vi "Decide Color Rank.vi"(11 "Numeric":dbl) -> (3 "Color Box":u32(colorbox))   [LabVIEW 2014]
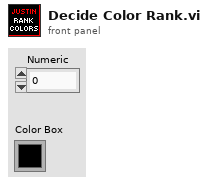
[diagram p1: front panel]
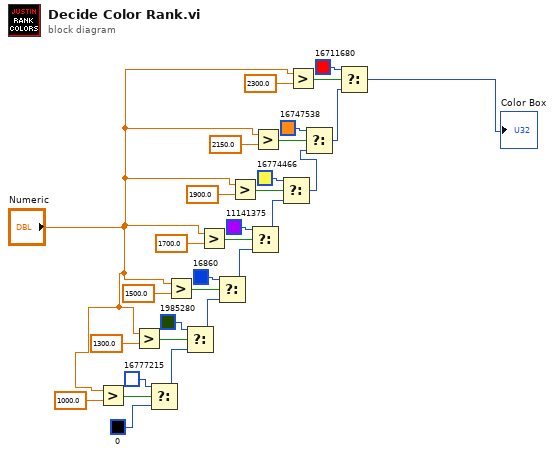
[diagram p0: block diagram]
diagram:
  n1 = Greater?(x="Numeric", y=1000.0) -> (0:w21:bool)
  n2 = Greater?(x="Numeric", y=1300.0) -> (0:w27:bool)
  n3 = Select(t=u32 16777215 ("Color Box"), s=w21, f=u32 0 ("Color Box")) -> (s? t:f=w20:u32)
  n4 = Greater?(x="Numeric", y=1500.0) -> (0:w29:bool)
  n5 = Select(t=u32 1985280 ("Color Box"), s=w27, f=w20) -> (s? t:f=w24:u32)
  n6 = Greater?(x="Numeric", y=1700.0) -> (0:w17:bool)
  n7 = Select(t=u32 16860 ("Color Box"), s=w29, f=w24) -> (s? t:f=w15:u32)
  n8 = Greater?(x="Numeric", y=1900.0) -> (0:w13:bool)
  n9 = Select(t=u32 11141375 ("Color Box"), s=w17, f=w15) -> (s? t:f=w11:u32)
  n10 = Greater?(x="Numeric", y=2150.0) -> (0:w9:bool)
  n11 = Select(t=u32 16774466 ("Color Box"), s=w13, f=w11) -> (s? t:f=w7:u32)
  n12 = Greater?(x="Numeric", y=2300.0) -> (0:w5:bool)
  n13 = Select(t=u32 16747538 ("Color Box"), s=w9, f=w7) -> (s? t:f=w3:u32)
  n14 = Select(t=u32 16711680 ("Color Box"), s=w5, f=w3) -> (s? t:f=→"Color Box":u32)
